vi "Get.vi"() -> ()   [LabVIEW 2012]
uses:
  Drive Global Data.vi
panel:
  in  "X All Power?":bool
  in  "Change Gear?":bool
  in  "Axis Y":dbl
  in  "Axis X":dbl
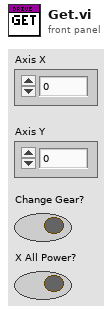
[diagram p1: front panel]
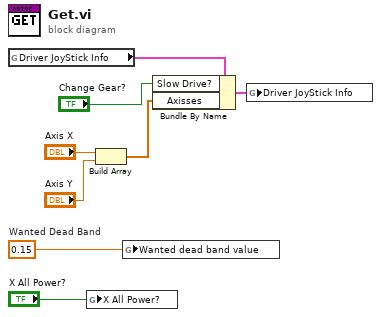
[diagram p0: block diagram]
diagram:
  w2 = 0.15  # Wanted Dead Band
  n1 = global read "Drive Global Data.vi" "Driver JoyStick Info"() -> (w8:cluster{"Slow Drive?":bool, "Axisses":dbl[]})
  n2 = global write "Drive Global Data.vi" "X All Power?"("X All Power?") -> ()
  n3 = Build Array("Axis X", "Axis Y") -> (w5:dbl[])
  n4 = global write "Drive Global Data.vi" "Wanted dead band value"(w2) -> ()
  n5 = Bundle By Name(cluster=w8, "Slow Drive?"="Change Gear?", "Axisses"=w5) -> (w3:cluster{"Slow Drive?":bool, "Axisses":dbl[]})
  n6 = global write "Drive Global Data.vi" "Driver JoyStick Info"(w3) -> ()
